vi "Velocity Variable.vi"() -> ()   [LabVIEW 2015]
panel:
  in  "Velocity":dbl
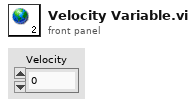
[diagram p1: front panel]
diagram:
